vi "Test.vi"() -> ()   [LabVIEW 2019]
panel:
  out "AngularPosition":T1
  out "device":T2
  in  "Test Trajectory Point":T3={"Position"={"Type"=enum."CARTESIAN_POSITION", "Delay"=0.0, "CartesianPosition"={"X"=0.025, "Y"=-0.3, "Z"=0.05, "ThetaX"=0.0, "ThetaY"=0.0, "ThetaZ"=0.0}, "Actuators"={"Actuator1"=0.0, "Actuator2"=0.0, "Actuator3"=0.0, "Actuator4"=0.0, "Actuator5"=0.0, "Actuator6"=0.0, "Actuator7"=0.0}, "HandMode"=enum."POSITION_MODE", "Fingers"={"Finger1"=6800.0, "Finger2"=6800.0, "Finger3"=0.0}}, "LimitationsActive"=FALSE, "SynchroType"=FALSE, "Limitations"={"speedParameter1"=0.0, "speedParameter2"=0.0, "speedParameter3"=0.0, "forceParameter1"=0.0, "forceParameter2"=0.0, "forceParameter3"=0.0, "accelerationParameter1"=0.0, "accelerationParameter2"=0.0, "accelerationParameter3"=0.0}}
  out "error out":errorcluster
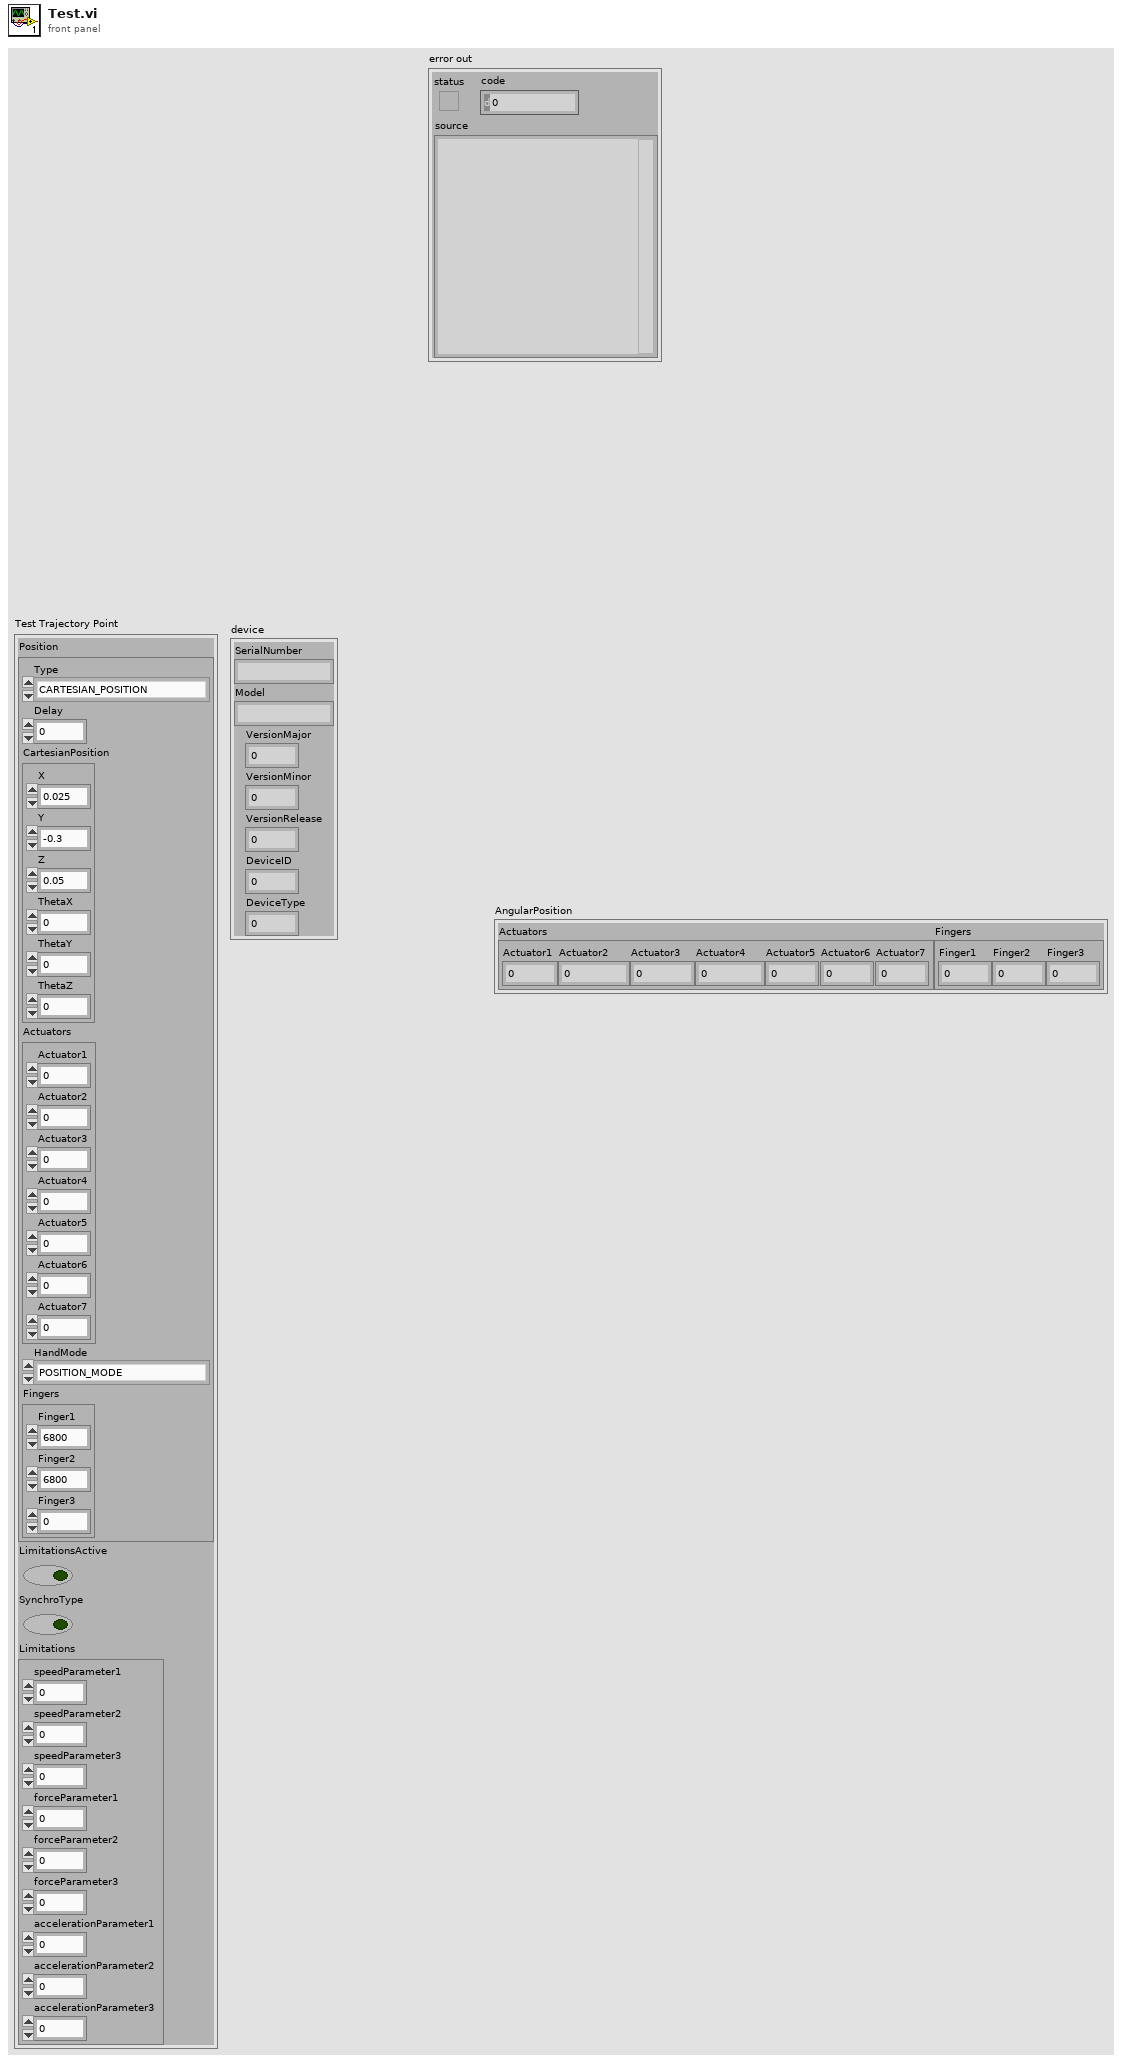
[diagram p1: front panel]
types:
  T1 = cluster{"Actuators":cluster{"Actuator1":sgl, "Actuator2":sgl, "Actuator3":sgl, "Actuator4":sgl, "Actuator5":sgl, "Actuator6":sgl, "Actuator7":sgl}, "Fingers":cluster{"Finger1":sgl, "Finger2":sgl, "Finger3":sgl}}
  T2 = cluster{"SerialNumber":string, "Model":string, "VersionMajor":i32, "VersionMinor":i32, "VersionRelease":i32, "DeviceID":i32, "DeviceType":i32}
  T3 = cluster{"Position":cluster{"Type":enum16{"NOMOVEMENT_POSITION", "CARTESIAN_POSITION", "ANGULAR_POSITION", "RETRACTED", "PREDEFINED1", "PREDEFINED2", "PREDEFINED3", "CARTESIAN_VELOCITY", "ANGULAR_VELOCITY", "PREDEFINED4", "PREDEFINED5", "ANY_TRAJECTORY", "TIME_DELAY"}, "Delay":sgl, "CartesianPosition":cluster{"X":sgl, "Y":sgl, "Z":sgl, "ThetaX":sgl, "ThetaY":sgl, "ThetaZ":sgl}, "Actuators":cluster{"Actuator1":sgl, "Actuator2":sgl, "Actuator3":sgl, "Actuator4":sgl, "Actuator5":sgl, "Actuator6":sgl, "Actuator7":sgl}, "HandMode":enum16{"HAND_NOMOVEMENT", "POSITION_MODE", "VELOCITY_MODE", "NO_FINGER", "ONE_FINGER", "TWO_FINGERS", "THREE_FINGERS"}, "Fingers":cluster{"Finger1":sgl, "Finger2":sgl, "Finger3":sgl}}, "LimitationsActive":bool, "SynchroType":bool, "Limitations":cluster{"speedParameter1":sgl, "speedParameter2":sgl, "speedParameter3":sgl, "forceParameter1":sgl, "forceParameter2":sgl, "forceParameter3":sgl, "accelerationParameter1":sgl, "accelerationParameter2":sgl, "accelerationParameter3":sgl}}
  T4 = cluster{"SerialNumber":string, "Model":string, "VersionMajor":i32, "VersionMinor":i32, "VersionRelease":i32, "DeviceID":i32, "DeviceType":i32}[]
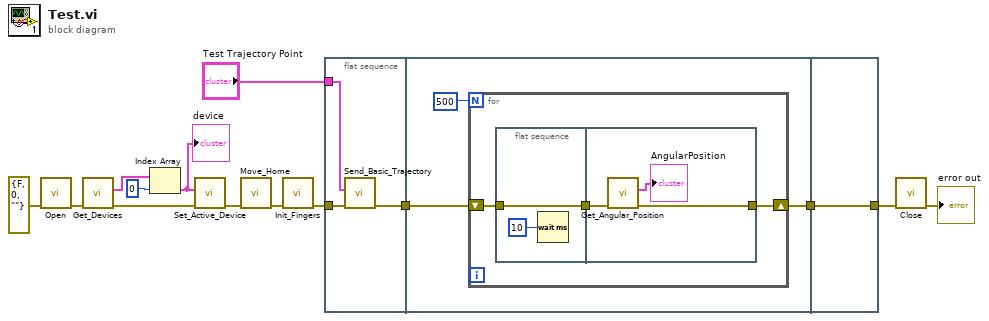
[diagram p0: block diagram]
diagram:
  n1 = call "Open.vi"("error in (no error)"=errorcluster {"status"=FALSE, "code"=0, "source"=""}) -> ("error out"=w13:errorcluster)  [unwired: 10 in]
  n2 = call "Get_Devices.vi"("error in (no error)"=w13) -> ("error out"=w8:errorcluster, "devices"=w11:T4)  [unwired: 9 in]
  n3 = Index Array(array=w11, index=0) -> (element=w9:T2)
  "device" <- w9
  n4 = call "Set_Active_Device.vi"("error in (no error)"=w8, "device"=w9) -> ("error out"=w7:errorcluster)  [unwired: 9 in]
  n5 = call "Move_Home.vi"("error in (no error)"=w7) -> ("error out"=w6:errorcluster)  [unwired: 10 in]
  n6 = call "Init_Fingers.vi"("error in (no error)"=w6) -> ("error out"=w5:errorcluster)  [unwired: 10 in]
  n7 = flat-sequence {
    tunnel: w5 -> [w17]
    tunnel: "Test Trajectory Point" -> [w15]
    tunnel: [w16] -> w2
    tunnel: w2 -> [w19]
    tunnel: [w20] -> w1
    tunnel: [w29] -> w4
    tunnel: w1 -> [w29]
    frame #0 {
      n8 = call "Send_Basic_Trajectory.vi"("error in (no error)"=w17, "TrajectoryPoint"=w15) -> ("error out"=w16:errorcluster)  [unwired: 9 in]
    }
    frame #1 {
      n9 = for {
        N: 500 -> [_]
        shift-right: [w22] -> w20
        shift-left: w19 -> [w21]
        n10 = flat-sequence {
          tunnel: w21 -> [w24]
          tunnel: [w24] -> w23
          tunnel: [w27] -> w22
          tunnel: w23 -> [w28]
          frame #0 {
            n11 = Wait (ms)(milliseconds to wait=u32 10) -> ()  [unwired: 1 out]
          }
          frame #1 {
            n12 = call "Get_Angular_Position.vi"("error in (no error)"=w28) -> ("error out"=w27:errorcluster, "AngularPosition"=→"AngularPosition":T1)  [unwired: 9 in]
          }
        }
      }
    }
    frame #2 {
    }
  }
  n13 = call "Close.vi"("error in (no error)"=w4) -> ("error out"=→"error out":errorcluster)  [unwired: 10 in]
